vi "myPICO_Open.vi"(6 "需要台数":u16, 7 "serials":u8[][](array[numeric]), 8 "错误输入（无错误）":errorcluster, 9 "触发阈值 (V)":dbl, 10 "触发方向":u16, 11 "示波器量程":u16) -> (2 "数组":T1(array[cluster]))   [LabVIEW 2024]
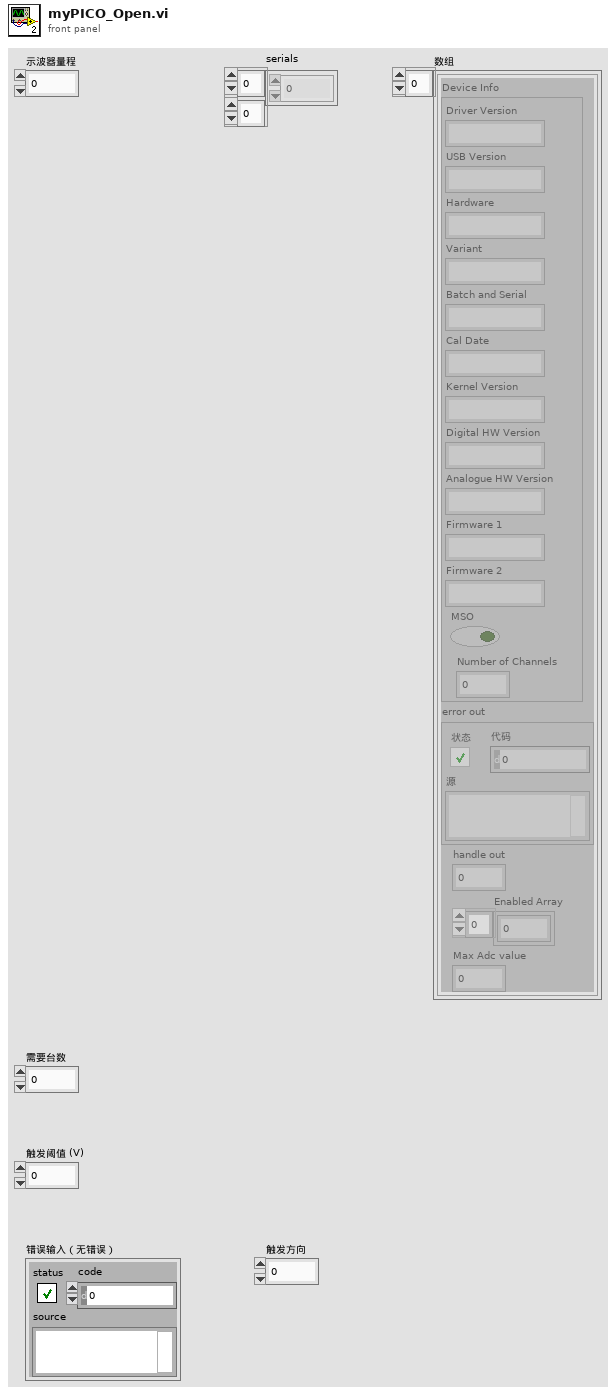
[diagram p1: front panel]
types:
  T1 = cluster{"Device Info":cluster{"Driver Version":string, "USB Version":string, "Hardware":string, "Variant":string, "Batch and Serial":string, "Cal Date":string, "Kernel Version":string, "Digital HW Version":string, "Analogue HW Version":string, "Firmware 1":string, "Firmware 2":string, "MSO":bool, "Number of Channels":i16}, "error out":errorcluster, "handle out":i16, "Enabled Array":i16[], "Max Adc value":i16}[]
  T2 = enum16{"Channel A", "Channel B", "Channel C", "Channel D", "Ext."}
  T3 = cluster{bool, "Trigger Source":enum16{"Channel A", "Channel B", "Channel C", "Channel D", "Ext."}, "触发阈值 (V)":dbl, "触发方向":u16, "Trigger Delay (samples)":u32, "Auto Trigger Time (ms)":i16}
  T4 = cluster{"Enabled":bool, "Coupling":i16, "示波器量程":u16, "Analogue Offset":sgl}
  T5 = cluster{"Driver Version":string, "USB Version":string, "Hardware":string, "Variant":string, "Batch and Serial":string, "Cal Date":string, "Kernel Version":string, "Digital HW Version":string, "Analogue HW Version":string, "Firmware 1":string, "Firmware 2":string, "MSO":bool, "Number of Channels":i16}
  T6 = cluster{"Device Info":cluster{"Driver Version":string, "USB Version":string, "Hardware":string, "Variant":string, "Batch and Serial":string, "Cal Date":string, "Kernel Version":string, "Digital HW Version":string, "Analogue HW Version":string, "Firmware 1":string, "Firmware 2":string, "MSO":bool, "Number of Channels":i16}, "error out":errorcluster, "handle out":i16, "Enabled Array":i16[], "Max Adc value":i16}
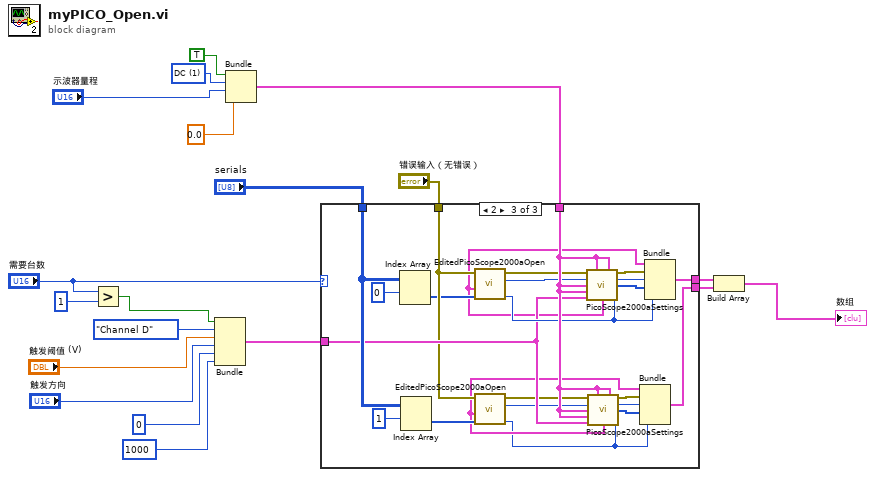
[diagram p0: block diagram]
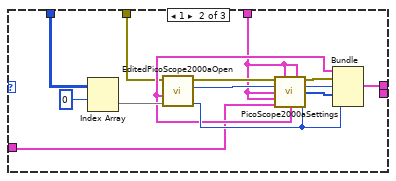
[diagram p3: hidden frame]
diagram:
  w12 = i16 1 items=["AC", "DC"] ("Coupling")
  n1 = Greater?(x="需要台数", y=1) -> (0:w2:bool)
  n2 = Bundle(w2, "Trigger Source"=T2."Channel D", "触发阈值 (V)"="触发阈值 (V)", "触发方向"="触发方向", "Trigger Delay (samples)"=u32 0, "Auto Trigger Time (ms)"=i16 1000) -> (w15:T3)  [unwired: 1 in]
  n3 = Bundle("Enabled"=TRUE, "Coupling"=w12, "示波器量程"="示波器量程", "Analogue Offset"=sgl 0.0) -> (w19:T4)  [unwired: 1 in]
  n4 = case shown="2" "需要台数" {
    tunnel: w19 -> [_ w23 w57]
    tunnel: [_ _ w56] -> w18
    tunnel: [_ w24 w55] -> w17
    tunnel: "serials" -> [_ w21 w50]
    tunnel: w15 -> [_ w20 w49]
    tunnel: "错误输入（无错误）" -> [_ w22 w48]
    frame 0, Default {
    }
    frame 1 {
      n5 = Index Array(array=w21, index (row)=0 ("索引 (行)")) -> (element=w28:u8[])  [unwired: 1 in]
      n6 = call "EditedPicoScope2000aOpen.vi"("serial"=w28, "error in (no error)"=w22) -> ("Max Adc value"=w31:i16, "handle"=w29:i16, "error out"=w27:errorcluster, "Device Info"=w25:T5)  [unwired: 2 in]
      n7 = call "PicoScope2000aSettings.vi"("error in"=w27, "Channel A Settings"=w23, "Channel B Settings"=w23, "handle in"=w29, "Channel C Settings"=w23, "Channel D Settings"=w23, "Trigger Settings"=w20, "Device Info"=w25, "Max_adc"=w31) -> ("error out"=w32:errorcluster, "handle out"=w33:i16, "Enabled Array"=w30:i16[])  [unwired: 4 in]
      n8 = Bundle("Device Info"=w25, "error out"=w32, "handle out"=w33, "Enabled Array"=w30, "Max Adc value"=w31) -> (w24:T6)  [unwired: 1 in]
    }
    frame 2 {
      n9 = Index Array(array=w50, index (row)=0 ("索引 (行)")) -> (element=w46:u8[])  [unwired: 1 in]
      n10 = Index Array(array=w50, index (row)=1 ("索引 (行)")) -> (element=w39:u8[])  [unwired: 1 in]
      n11 = call "EditedPicoScope2000aOpen.vi"("serial"=w46, "error in (no error)"=w48) -> ("Max Adc value"=w52:i16, "handle"=w47:i16, "error out"=w45:errorcluster, "Device Info"=w43:T5)  [unwired: 2 in]
      n12 = call "EditedPicoScope2000aOpen.vi"("serial"=w39, "error in (no error)"=w48) -> ("Max Adc value"=w34:i16, "handle"=w41:i16, "error out"=w42:errorcluster, "Device Info"=w38:T5)  [unwired: 2 in]
      n13 = call "PicoScope2000aSettings.vi"("error in"=w45, "Channel A Settings"=w57, "Channel B Settings"=w57, "handle in"=w47, "Channel C Settings"=w57, "Channel D Settings"=w57, "Trigger Settings"=w49, "Device Info"=w43, "Max_adc"=w52) -> ("error out"=w53:errorcluster, "handle out"=w54:i16, "Enabled Array"=w51:i16[])  [unwired: 4 in]
      n14 = call "PicoScope2000aSettings.vi"("error in"=w42, "Channel A Settings"=w57, "Channel B Settings"=w57, "handle in"=w41, "Channel C Settings"=w57, "Channel D Settings"=w57, "Trigger Settings"=w49, "Device Info"=w38, "Max_adc"=w34) -> ("error out"=w37:errorcluster, "handle out"=w36:i16, "Enabled Array"=w35:i16[])  [unwired: 4 in]
      n15 = Bundle("Device Info"=w38, "error out"=w37, "handle out"=w36, "Enabled Array"=w35, "Max Adc value"=w34) -> (w56:T6)  [unwired: 1 in]
      n16 = Bundle("Device Info"=w43, "error out"=w53, "handle out"=w54, "Enabled Array"=w51, "Max Adc value"=w52) -> (w55:T6)  [unwired: 1 in]
    }
  }
  n17 = Build Array(w17, w18) -> (→"数组":T1)
